vi "CI Project UI.vi"() -> ()   [LabVIEW 2014, in "CI Project.lvclass"]
uses:
  CI Project.lvclass
  <vilib>/ni/Configuration Framework/Node/NodeRef.ctl
  <vilib>/ni/Configuration Framework/Node/NISE_CEF_Node.lvclass
  <vilib>/ni/AMC/Message Queue.ctl
  <vilib>/ni/AMC/Message.ctl
  <vilib>/ni/Tools/Keyed Array/KeyedArray.ctl
  <vilib>/ni/Configuration Framework/Node/UserEventRef.ctl
  <vilib>/ni/Configuration Framework/Controls/EventCluster.ctl
  CI Project.lvclass/CI Project.ctl
  Build Job/Build Job.lvclass/Build Job.ctl
  <vilib>/ni/AMC/Create Single Message.vi
  <vilib>/ni/AMC/Update Message Routing Info.vi
  <vilib>/ni/AMC/Send Message.vi
  <vilib>/ni/AMC/AMC.lvlib
  Build Job/Build Job.lvclass
  <vilib>/ni/Tools/Keyed Array/Tools_KeyedArray.lvlib
  <vilib>/ni/Configuration Framework/NISE_CEF_TreeControl.lvlib
panel:
  in  "Root Workspace Folder":path=path "C:/Projects/LabVIEW Continuous Integration/LabVIEW Continuous Integration.lvproj"
  in  "Description":string="brandyn.adderley@ni.com"
  in  "user event":T1
  in  "main queue":T2
  in  "node ref":T3
  in  "Hostname":string caption="Jenkins Hostname(IP Address:Port Number)"
  in  "Project Name":string="LabVIEW Test"
  in  "Artifact Days":i32=15 caption="How many days to Artifact?"
  in  "Notification":string="brandyn.adderley@ni.com" caption="Notification (Separate by Space)"
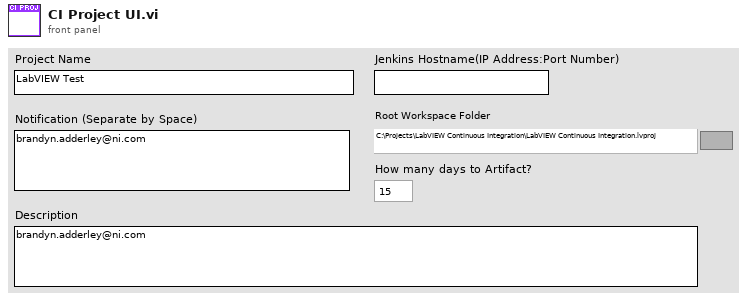
[diagram p1: front panel]
types:
  T1 = typedef "NISE_CEF_Node.lvclass/UserEventRef.ctl" = refnum<user-event>
  T2 = typedef "AMC.lvlib/Message Queue.ctl" = refnum<queue>
  T3 = typedef "NISE_CEF_Node.lvclass/NodeRef.ctl" = refnum<data-value>
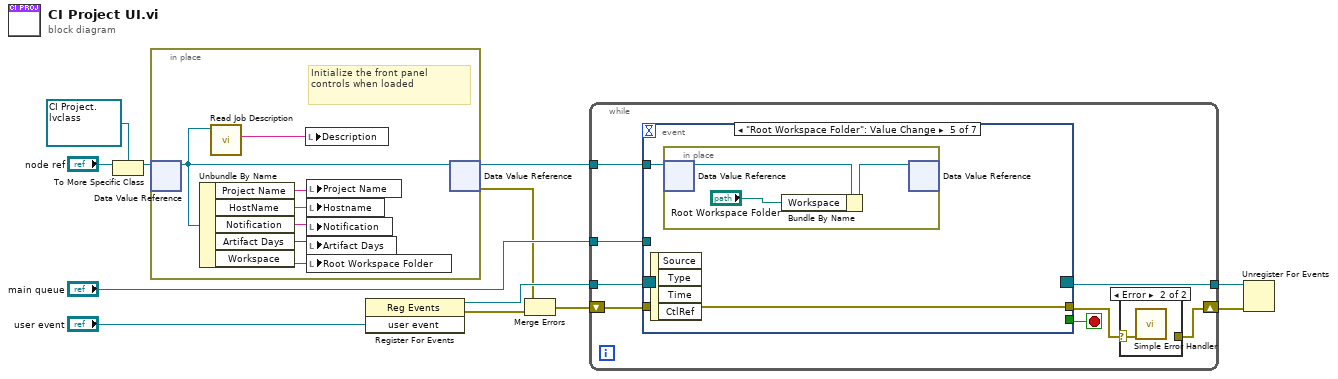
[diagram p0: block diagram]
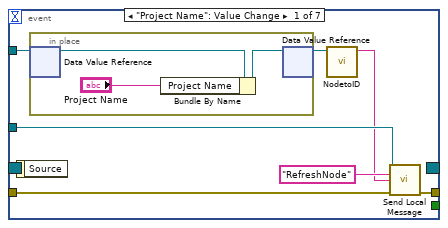
[diagram p3: hidden frame]
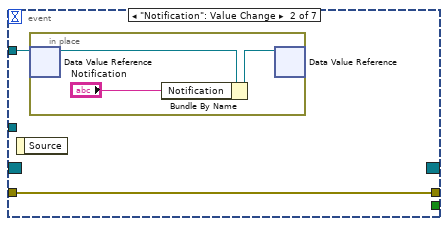
[diagram p4: hidden frame]
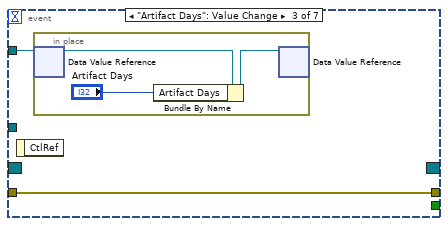
[diagram p5: hidden frame]
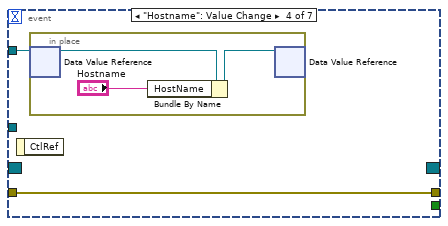
[diagram p6: hidden frame]
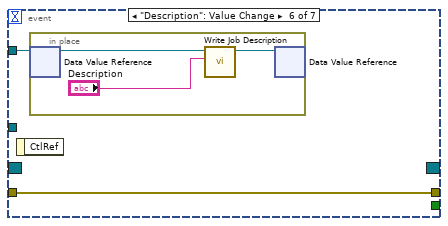
[diagram p7: hidden frame]
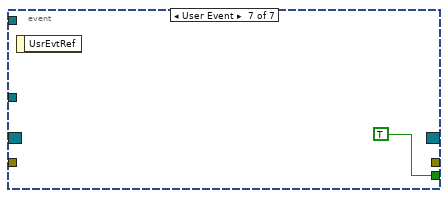
[diagram p8: hidden frame]
diagram:
  n1 = To More Specific Class(target class=refnum<data-value> refnum ("data value reference"), reference="node ref") -> (specific class reference=w6:refnum<data-value>)  [unwired: 1 in, 1 out]
  n2 = in-place {
    # "Initialize the front panel controls when loaded"
    n3 = in-place-dvr #1(w6) -> (w15:refnum<class "CI Project.lvclass">)  [unwired: 1 out]
    n4 = Unbundle By Name(w15) -> ("Project Name"=w19:string, "HostName"=w18:string, "Notification"=w17:string, "Artifact Days"=w16:i32, "Workspace"=w13:path)
    n5 = call-dynamic "Read Job Description.vi"("Build Job in"=w15) -> ("Job Description"=w14:string)  [unwired: 10 in]
    n6 = local write "Description"(w14) -> ()
    n7 = local write "Project Name"(w19) -> ()
    n8 = local write "Hostname"(w18) -> ()
    n9 = local write "Notification"(w17) -> ()
    n10 = local write "Artifact Days"(w16) -> ()
    n11 = local write "Root Workspace Folder"(w13) -> ()
    n12 = in-place-dvr #1(w15) -> (w1:refnum<data-value>, w3:errorcluster)
  }
  n13 = register-events("user event") -> (reference out=w10:refnum<event-registration>, error out=w4:errorcluster)  [unwired: 2 in]
  n14 = Merge Errors(w3, w4) -> (w2:errorcluster)
  n15 = while {
    tunnel: w1 -> [w27]
    tunnel: "main queue" -> [w26]
    tunnel: w10 -> [w25]
    tunnel: [w24] -> w9
    shift-right: [w20] -> w8
    shift-left: w2 -> [w23]
    stop <- w22 stop-if-true
    n16 = event shown="[4] \"Root Workspace Folder\": Value Change" {
      selector: w25 -> [_ _ _ _ _ _ _]
      dyn-events: [_ _ _ _ _ _ _] -> w24
      timeout: _ -> [_ _ _ _ _ _ _]
      tunnel: w27 -> [w34 w41 w46 w51 w56 w61 _]
      tunnel: w26 -> [w35 _ _ _ _ _ _]
      tunnel: [_ _ _ _ _ _ TRUE] -> w22
      tunnel: [w32 w40 w45 w50 w55 w60 _] -> w21
      tunnel: w23 -> [w31 w40 w45 w50 w55 w60 _]
      event "Project Name": Value Change {
        n17 = event-data() -> ()  [unwired: 1 in, 1 out]
        n18 = in-place {
          n19 = in-place-dvr #2(w34) -> (w39:refnum<class "CI Project.lvclass">)  [unwired: 1 out]
          n20 = Bundle By Name(cluster=w39, "Project Name"="Project Name") -> (w38:refnum<class "CI Project.lvclass">)
          n21 = in-place-dvr #2(w38) -> (w30:refnum<data-value>)  [unwired: 1 out]
        }
        n22 = call <vilib>:"NodetoID.vi"("node ref"=w30) -> ("ID"=w33:string)  [unwired: 9 in, 1 out]
        n23 = call <vilib>:"Send Local Message.vi"("message queue in"=w35, "message name"="RefreshNode" ("Message Name"), "message value"=w33, "error in"=w31) -> ("error out"=w32:errorcluster)  [unwired: 9 in, 2 out]
      }
      event "Notification": Value Change {
        n24 = event-data() -> ()  [unwired: 1 in, 1 out]
        n25 = in-place {
          n26 = in-place-dvr #3(w41) -> (w44:refnum<class "CI Project.lvclass">)  [unwired: 1 out]
          n27 = Bundle By Name(cluster=w44, "Notification"="Notification") -> (w43:refnum<class "CI Project.lvclass">)
          n28 = in-place-dvr #3(w43) -> ()  [unwired: 2 out]
        }
      }
      event "Artifact Days": Value Change {
        n29 = event-data() -> ()  [unwired: 1 in, 1 out]
        n30 = in-place {
          n31 = in-place-dvr #4(w46) -> (w49:refnum<class "CI Project.lvclass">)  [unwired: 1 out]
          n32 = Bundle By Name(cluster=w49, "Artifact Days"="Artifact Days") -> (w48:refnum<class "CI Project.lvclass">)
          n33 = in-place-dvr #4(w48) -> ()  [unwired: 2 out]
        }
      }
      event "Hostname": Value Change {
        n34 = event-data() -> ()  [unwired: 1 in, 1 out]
        n35 = in-place {
          n36 = in-place-dvr #5(w51) -> (w54:refnum<class "CI Project.lvclass">)  [unwired: 1 out]
          n37 = Bundle By Name(cluster=w54, "HostName"="Hostname") -> (w53:refnum<class "CI Project.lvclass">)
          n38 = in-place-dvr #5(w53) -> ()  [unwired: 2 out]
        }
      }
      event "Root Workspace Folder": Value Change {
        n39 = event-data() -> ()  [unwired: 1 in, 4 out]
        n40 = in-place {
          n41 = in-place-dvr #6(w56) -> (w59:refnum<class "CI Project.lvclass">)  [unwired: 1 out]
          n42 = Bundle By Name(cluster=w59, "Workspace"="Root Workspace Folder") -> (w58:refnum<class "CI Project.lvclass">)
          n43 = in-place-dvr #6(w58) -> ()  [unwired: 2 out]
        }
      }
      event "Description": Value Change {
        n44 = event-data() -> ()  [unwired: 1 in, 1 out]
        n45 = in-place {
          n46 = in-place-dvr #7(w61) -> (w64:refnum<class "CI Project.lvclass">)  [unwired: 1 out]
          n47 = call "Write Job Description.vi"("Job Description"="Description", "Build Job in"=w64) -> ("Build Job out"=w63:refnum<class "CI Project.lvclass">)  [unwired: 9 in]
          n48 = in-place-dvr #7(w63) -> ()  [unwired: 2 out]
        }
      }
      event User Event {
        n49 = event-data() -> ()  [unwired: 1 in, 1 out]
      }
    }
    n50 = case shown="Error" w21 {
      selector: w21 -> [w28 w29]
      tunnel: [w28 _] -> w20
      frame No Error {
      }
      frame Error {
        n51 = call <vilib>:"Simple Error Handler.vi"("error in (no error)"=w29) -> ()  [unwired: 4 in, 5 out]
      }
    }
  }
  n52 = Unregister For Events(event registration refnum=w9, error in=w8) -> ()  [unwired: 1 out]
